vi "Sinusoidal.vi"   [LabVIEW 2017]
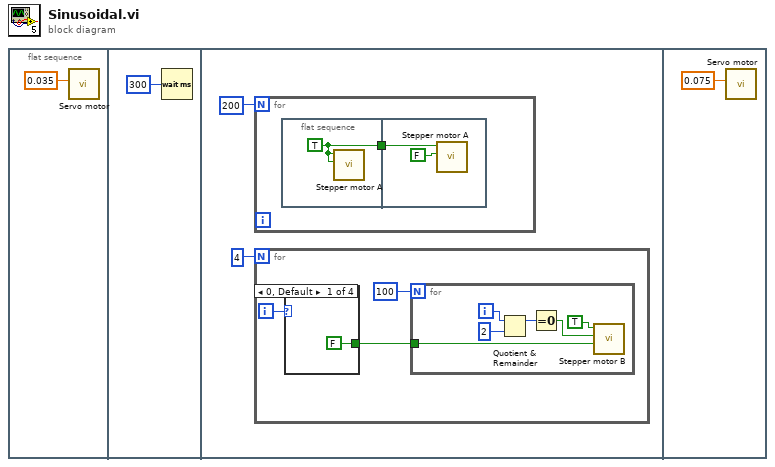
[diagram p0: block diagram]
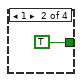
[diagram p2: hidden frame]
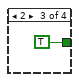
[diagram p3: hidden frame]
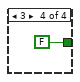
[diagram p4: hidden frame]
diagram:
  n1 = flat-sequence {
    frame #0 {
      n2 = call "Servo motor.vi"("Duty Cycle"=0.035) -> ()  [unwired: 9 in, 2 out]
    }
    frame #1 {
      n3 = Wait (ms)(milliseconds to wait=u32 300) -> ()  [unwired: 1 out]
    }
    frame #2 {
      n4 = for {
        N: 200 ("Numeric") -> [_]
        n5 = flat-sequence {
          tunnel: [w19] -> w18
          tunnel: w18 -> [w21]
          frame #0 {
            w19 = TRUE ("Enable (C/DIO2 (DIO2))")
            n6 = call "Stepper motor A.vi"("Step (C/DIO3 (DIO3))"=w19, "Enable (C/DIO2 (DIO2))"=w19) -> ()  [unwired: 9 in, 1 out]
          }
          frame #1 {
            n7 = call "Stepper motor A.vi"("Step (C/DIO3 (DIO3))"=FALSE, "Enable (C/DIO2 (DIO2))"=w21) -> ()  [unwired: 9 in, 1 out]
          }
        }
      }
      n8 = for {
        N: 4 -> [_]
        i -> [w6]
        n9 = case shown="0, Default" w6 {
          tunnel: [FALSE TRUE TRUE FALSE] -> w5
          frame 0, Default {
          }
          frame 1 {
          }
          frame 2 {
          }
          frame 3 {
          }
        }
        n10 = for {
          N: 100 -> [_]
          tunnel: w5 -> [w12]
          i -> [w13]
          n11 = Quotient & Remainder(x=w13, y=2) -> (x-y*floor(x/y)=w15:i32)  [unwired: 1 out]
          n12 = Equal To 0?(x=w15) -> (x = 0?=w14:bool)
          n13 = call "Stepper motor B.vi"("Direction (A/DIO5 (Pin 21))"=w12, "Step (A/DIO4 (Pin 19))"=w14, "Enable (A/DIO0 (Pin 11))"=TRUE ("Enable (C/DIO2 (DIO2))")) -> ()  [unwired: 7 in, 2 out]
        }
      }
    }
    frame #3 {
      n14 = call "Servo motor.vi"("Duty Cycle"=0.075) -> ()  [unwired: 9 in, 2 out]
    }
  }
